vi "DCIMG File Names.vi"(9 "Camera Type":T1, 10 "Channel Names":string[](array[string]), 11 "TIFF File Path":path) -> (3 "DCIMG Files":path[](array[path]))   [LabVIEW 2022 SP3]
uses:
  Type Defs/Camera Type.ctl
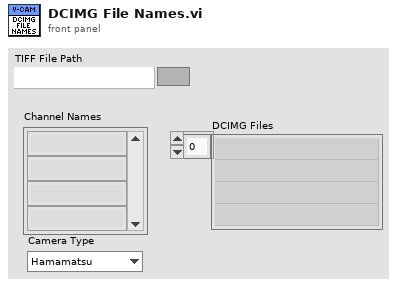
[diagram p1: front panel]
types:
  T1 = typedef "Camera Type.ctl" = enum16{"Hamamatsu", "Andor", "Photometrics"}
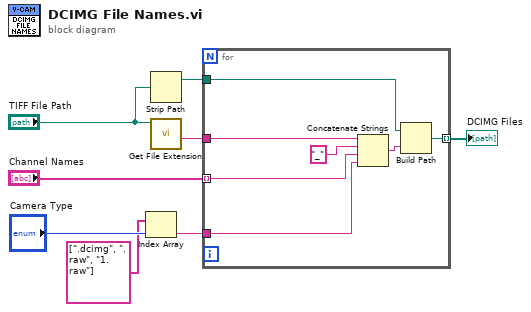
[diagram p0: block diagram]
diagram:
  n1 = Index Array(array=string[] [".dcimg", ".raw", "1.raw"], index="Camera Type") -> (element=w2:string)
  n2 = Strip Path(path="TIFF File Path") -> (stripped path=w6:path)  [unwired: 1 out]
  n3 = call <vilib>:"Get File Extension.vi"("file"="TIFF File Path") -> ("filename without extension"=w7:string)  [unwired: 6 in, 4 out]
  n4 = for {
    tunnel: w7 -> [w15]
    tunnel: w6 -> [w13]
    tunnel: [w12] -> w5 mode=indexing
    tunnel: "Channel Names" -> [w11] mode=indexing
    tunnel: w2 -> [w9]
    n5 = Concatenate Strings(w15, "_" ("string"), w11, w9) -> (w14:string)
    n6 = Build Path(base path=w13, name or relative path=w14) -> (appended path=w12:path)
  }
  "DCIMG Files" <- w5
